vi "DAQ timeControlParameters.vi"(3 "tiempo (ms)":dbl, 5 "DAQ Device IN":T1) -> (1 "#samples":u32, 2 "Time Control Parameters":cluster{"# samples":u32, "tiempos (ms)":dbl})   [LabVIEW 2010]
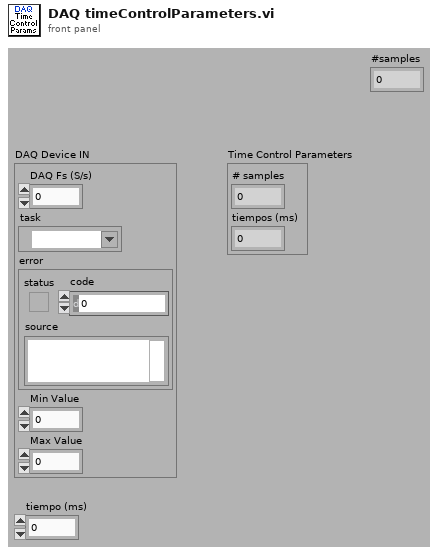
[diagram p1: front panel]
types:
  T1 = cluster{"DAQ Fs (S/s)":dbl, "task":refnum<k21>, "error":errorcluster, "Min Value":dbl, "Max Value":dbl}
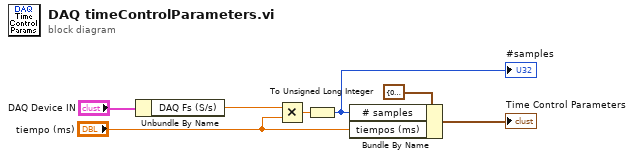
[diagram p0: block diagram]
diagram:
  n1 = Unbundle By Name("DAQ Device IN") -> ("DAQ Fs (S/s)"=w7:dbl)
  n2 = Multiply(x=w7, y="tiempo (ms)") -> (x*y=w3:dbl)
  n3 = To Unsigned Long Integer(number=w3) -> (unsigned 32bit integer=w4:u32)
  "#samples" <- w4
  n4 = Bundle By Name(cluster=cluster{"# samples":u32, "tiempos (ms)":dbl} {"# samples"=0, "tiempos (ms)"=0.0} ("Time Control Parameters"), "# samples"=w4, "tiempos (ms)"="tiempo (ms)") -> (→"Time Control Parameters":cluster{"# samples":u32, "tiempos (ms)":dbl})
